vi "Launch N DUTs.vi"() -> ()   [LabVIEW 2023]
uses:
  DUT Sample/typedefs/DUT HW Resources.ctl
  DUT Sample/DUT Sample.lvclass
panel:
  in  "DUTs Config":T1[](array[typedef])=[{"CAN Interface"="CAN2", "CAN Termination"=TRUE, "Digital Counter"="PXI1Slot8/ctr0", "DO Terminals"=["/PXI1Slot8/PFI0", "/PXI1Slot8/PFI1", "/PXI1Slot8/PFI2", "/PXI1Slot8/PFI3", "/PXI1Slot8/PFI4", "/PXI1Slot8/PFI5", "/PXI1Slot8/PFI6", "/PXI1Slot8/PFI7"]}, {"CAN Interface"="CAN4", "CAN Termination"=TRUE, "Digital Counter"="PXI1Slot8/ctr1", "DO Terminals"=["/PXI1Slot8/PFI2", "/PXI1Slot8/PFI3", "/PXI1Slot8/PFI2", "/PXI1Slot8/PFI3", "/PXI1Slot8/PFI4", "/PXI1Slot8/PFI5", "/PXI1Slot8/PFI6", "/PXI1Slot8/PFI7"]}, {"CAN Interface"="CAN6", "CAN Termination"=TRUE, "Digital Counter"="PXI1Slot8/ctr2", "DO Terminals"=["/PXI1Slot8/PFI4", "/PXI1Slot8/PFI5", "/PXI1Slot8/PFI2", "/PXI1Slot8/PFI3", "/PXI1Slot8/PFI4", "/PXI1Slot8/PFI5", "/PXI1Slot8/PFI6", "/PXI1Slot8/PFI7"]}]
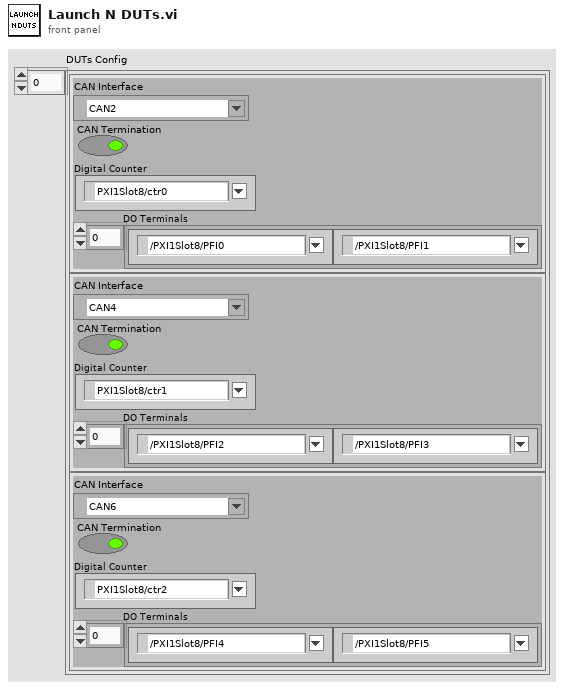
[diagram p1: front panel]
types:
  T1 = typedef "DUT Sample.lvclass/DUT HW Resources.ctl" = cluster{"CAN Interface":refnum<k21>, "CAN Termination":bool, "Digital Counter":tag, "DO Terminals":tag[]}
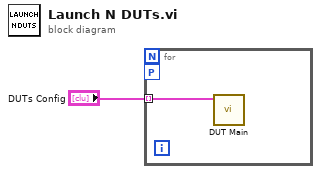
[diagram p0: block diagram]
diagram:
  n1 = for {
    workers-P: _ -> [_]
    tunnel: "DUTs Config" -> [w2] mode=indexing
    n2 = call "DUT Main.vi"("DUT HW Resources"=w2) -> ()  [unwired: 11 in]
  }
